vi "SEA_9811_Read.vi"(8 "error in (no error)":errorcluster, 11 "SEA9811_RT_data in":T2 {"Tx"."Tx Refs (Data,Trig)"."Data Reference" format="%.0x"}) -> (0 "error out":errorcluster, 1 "Receiver Status Register (RSR)":T1={"RSR0: FIFO channel 0 empty"=TRUE, "RSR1: FIFO channel 1 empty"=TRUE, "RSR2: FIFO channel 2 empty"=TRUE, "RSR3: FIFO channel 3 empty"=TRUE, "RSR4: FIFO channel 4 empty"=TRUE, "RSR5: FIFO channel 5 empty"=TRUE, "RSR6: FIFO channel 6 empty"=TRUE, "RSR7: FIFO channel 7 empty"=TRUE, "RSR8: FIFO channel 0 full"=FALSE, "RSR9: FIFO channel 1 full"=FALSE, "RSR10: FIFO channel 2 full"=FALSE, "RSR11: FIFO channel 3 full"=FALSE, "RSR12: FIFO channel 4 full"=FALSE, "RSR13: FIFO channel 5 full"=FALSE, "RSR14: FIFO channel 6 full"=FALSE, "RSR15: FIFO channel 7 full"=FALSE}, 3 "SEA9811_RT_data out":T2 {"Tx"."Tx Refs (Data,Trig)"."Data Reference" format="%.0x"}, 5 "DMA Overflow":bool)   [LabVIEW 2012]
doc: "Read words from FPGA, process and sync clock"
uses:
  Typdefs/SEA9811_RT_data_cluster.ctl
  <userlib>/_FPGA Interface Advanced Tools/FPGA Interface Base/FPGA Interface Base.lvclass
  Typdefs/FPGA ref.ctl
  Typdefs/channel.ctl
  Typdefs/received word.ctl
  Typdefs/SEA9811_FPGA_FP_Addresses.ctl
  <vilib>/NI Veristand/Custom Device API/Block Data Reference.ctl
  <vilib>/NI Veristand/Custom Device API/Data Reference.ctl
  FPGA/SEA-9811_ReceiverAndTransmitter/SubVIs/SEA-9811_ReceiverAndTransmitter_RSR.ctl
  <userlib>/_FPGA Interface Advanced Tools/FPGA Interface Wrapper/NiFPGA Read - U32.vi
  <userlib>/_FPGA Interface Advanced Tools/FPGA Interface Wrapper/NiFPGA Read - Boolean.vi
  <userlib>/_FPGA Interface Advanced Tools/FPGA Interface Wrapper/NiFPGA Read FIFO - U64.vi
  <userlib>/_FPGA Interface Advanced Tools/FPGA Interface Wrapper/NiFPGA Read - U16.vi
  <userlib>/_FPGA Interface Advanced Tools/FPGA Interface Wrapper/FPGA Interface Wrapper.lvlib
  <vilib>/NI Veristand/Custom Device API/Custom Device API.lvlib
panel:
  out "Elements Remaining":u32
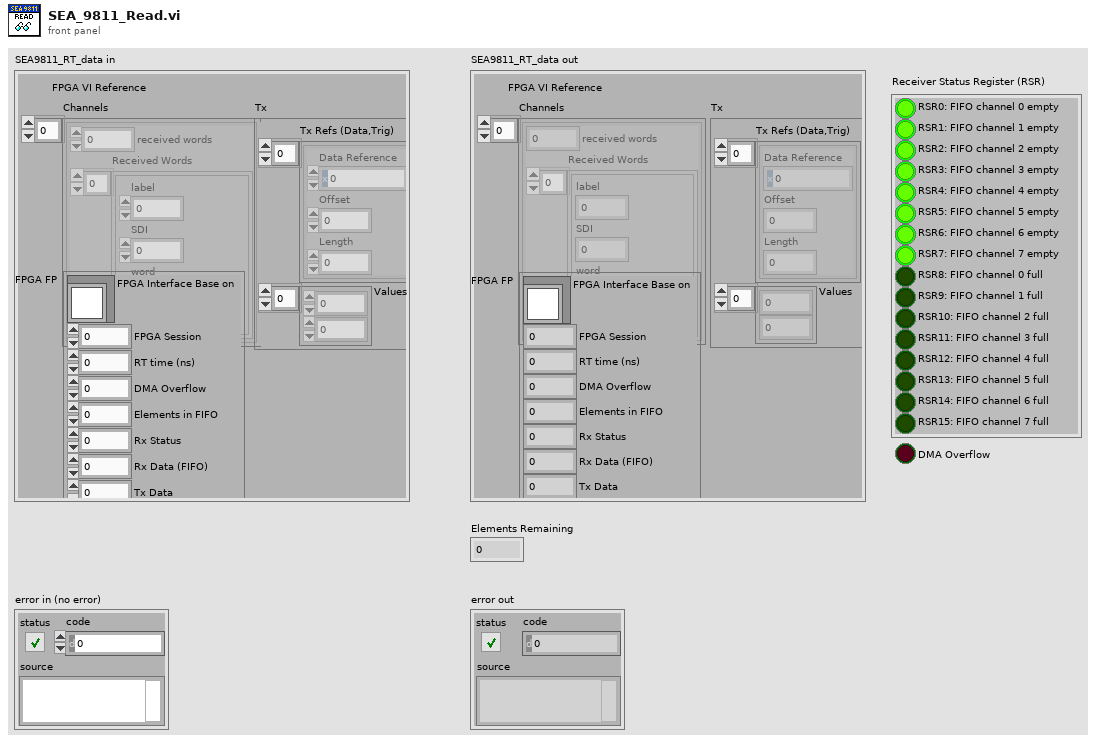
[diagram p1: front panel]
types:
  T1 = typedef "SEA-9811_ReceiverAndTransmitter_RSR.ctl" = cluster{"RSR0: FIFO channel 0 empty":bool, "RSR1: FIFO channel 1 empty":bool, "RSR2: FIFO channel 2 empty":bool, "RSR3: FIFO channel 3 empty":bool, "RSR4: FIFO channel 4 empty":bool, "RSR5: FIFO channel 5 empty":bool, "RSR6: FIFO channel 6 empty":bool, "RSR7: FIFO channel 7 empty":bool, "RSR8: FIFO channel 0 full":bool, "RSR9: FIFO channel 1 full":bool, "RSR10: FIFO channel 2 full":bool, "RSR11: FIFO channel 3 full":bool, "RSR12: FIFO channel 4 full":bool, "RSR13: FIFO channel 5 full":bool, "RSR14: FIFO channel 6 full":bool, "RSR15: FIFO channel 7 full":bool}
  T2 = typedef "SEA9811_RT_data_cluster.ctl" = cluster{"FPGA VI Reference":T3, "Channels":T4[], "FPGA FP":T6, "Tx":cluster{"Tx Refs (Data,Trig)":T7[], "Values":dbl[]}}
  T3 = typedef "FPGA ref.ctl" = refnum<k20>
  T4 = typedef "channel.ctl" = cluster{"received words":u32, "Received Words":T5[]}
  T5 = typedef "received word.ctl" = cluster{"label":u8, "SDI":u8, "word":u32, "timestamp":dbl}
  T6 = typedef "SEA9811_FPGA_FP_Addresses.ctl" = cluster{"FPGA Interface Base on":refnum<class "FPGA Interface Base.lvclass">, "FPGA Session":u32, "RT time (ns)":u32, "DMA Overflow":u32, "Elements in FIFO":u32, "Rx Status":u32, "Rx Data (FIFO)":u32, "Tx Data":u32, "Transmit Data":u32}
  T7 = typedef "Custom Device API.lvlib/Block Data Reference.ctl" = cluster{"Data Reference":T8, "Offset":i32, "Length":i32}
  T8 = typedef "Custom Device API.lvlib/Data Reference.ctl" = i32
  T9 = cluster{"Boolean array[0]":bool, "Boolean array[1]":bool, "Boolean array[2]":bool, "Boolean array[3]":bool, "Boolean array[4]":bool, "Boolean array[5]":bool, "Boolean array[6]":bool, "Boolean array[7]":bool, "Boolean array[8]":bool, "Boolean array[9]":bool, "Boolean array[10]":bool, "Boolean array[11]":bool, "Boolean array[12]":bool, "Boolean array[13]":bool, "Boolean array[14]":bool, "Boolean array[15]":bool}
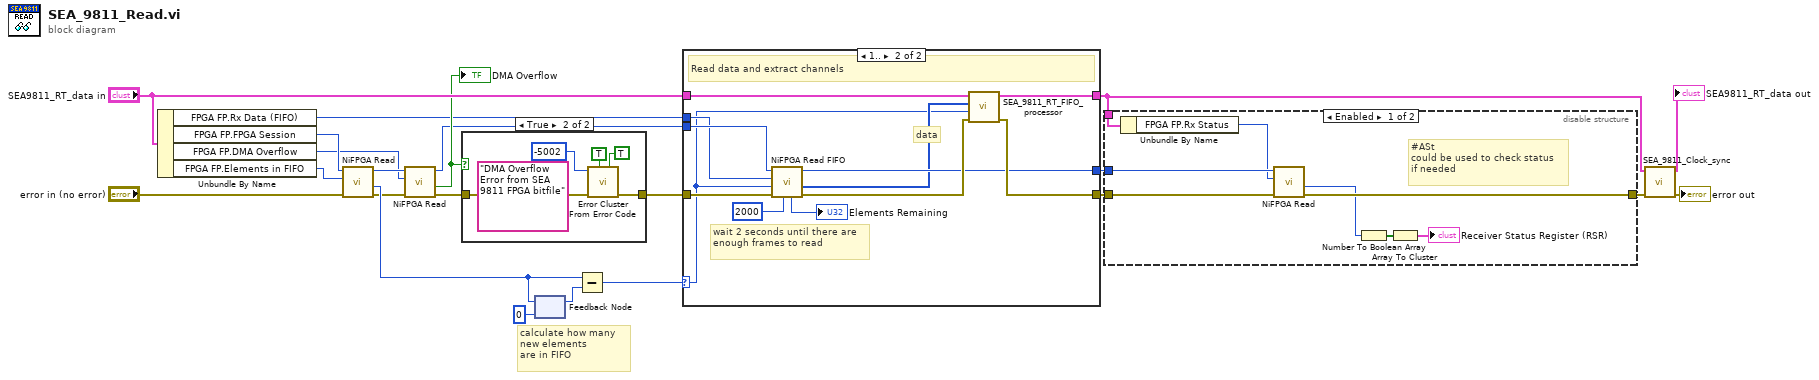
[diagram p0: block diagram]
diagram:
  # "calculate how many \nnew elements \nare in FIFO"
  n1 = Unbundle By Name("SEA9811_RT_data in") -> ("FPGA FP.Rx Data (FIFO)"=w6:u32, "FPGA FP.FPGA Session"=w17:u32, "FPGA FP.DMA Overflow"=w11:u32, "FPGA FP.Elements in FIFO"=w16:u32)
  n2 = call-poly <userlib>:"NiFPGA Read.vi"("error in (no error)"="error in (no error)", "Indicator"=w16, "Session"=w17) -> ("error out"=w12:errorcluster, "Value"=w14:u32, "Session Out"=w13:u32)  [unwired: 6 in]
  n3 = call-poly <userlib>:"NiFPGA Read.vi"("error in (no error)"=w12, "Indicator"=w11, "Session"=w13) -> ("error out"=w10:errorcluster, "Boolean"=w8:bool, "Session Out"=w7:u32)  [unwired: 6 in]
  "DMA Overflow" <- w8
  n4 = case shown="True" w8 {
    tunnel: w10 -> [w23 w29]
    tunnel: [w23 w28] -> w9
    frame False {
    }
    frame True {
      n5 = call <vilib>:"Error Cluster From Error Code.vi"("is warning? (False)"=TRUE, "show call chain? (False)"=TRUE, "error in (no error)"=w29, "error message (\"\")"="DMA Overflow Error from SEA 9811 FPGA bitfile" ("error message (\"\")"), "error code (0)"=-5002) -> ("error out"=w28:errorcluster)  [unwired: 4 in]
    }
  }
  n6 = feedback-in #1(w14) -> ()
  n7 = feedback #1(u32 0 ("Elements in FIFO")) -> (w22:u32)
  n8 = Subtract(x=w14, y=w22) -> (x-y=w1:u32)
  n9 = case shown="1.." w1 {
    selector: w1 -> [_ w33]
    tunnel: [w31 w42] -> w4
    tunnel: "SEA9811_RT_data in" -> [w32 w44]
    tunnel: [w32 w43] -> w5
    tunnel: w9 -> [w31 w40]
    tunnel: w7 -> [w30 w41]
    tunnel: w6 -> [_ w38]
    tunnel: [w30 w37] -> w2
    frame Default {
      # "not enough data to read"
    }
    frame 1.. {
      # "wait 2 seconds until there are enough frames to read"
      # "data"
      # "Read data and extract channels"
      n10 = call-poly <userlib>:"NiFPGA Read FIFO.vi"("Timeout"=u32 2000, "error in (no error)"=w40, "Number of Elements"=w33, "FIFO"=w38, "Session"=w41) -> ("error out"=w39:errorcluster, "Data"=w34:u64[], "Session Out"=w37:u32, "Elements Remaining"=→"Elements Remaining":u32)  [unwired: 3 in]
      n11 = call "SEA_9811_RT_FIFO_processor.vi"("error in (no error)"=w39, "Number of Elements"=w33, "9811 Data in"=w34, "SEA9811_RT_data in"=w44) -> ("error out"=w42:errorcluster, "SEA9811_RT_data out"=w43:T2)  [unwired: 6 in]
    }
  }
  n12 = disable-structure shown="Enabled" {
    disable-tunnel: w5 -> [w50 _]
    disable-tunnel: w4 -> [w49 w53]
    disable-tunnel: [w48 w53] -> w3
    disable-tunnel: w2 -> [w47 _]
    frame Enabled {
      # "#ASt\ncould be used to check status\nif needed"
      n13 = Unbundle By Name(w50) -> ("FPGA FP.Rx Status"=w46:u32)
      n14 = call-poly <userlib>:"NiFPGA Read.vi"("error in (no error)"=w49, "Indicator"=w46, "Session"=w47) -> ("error out"=w48:errorcluster, "Value"=w45:u16)  [unwired: 6 in, 1 out]
      n15 = Number To Boolean Array(number=w45) -> (Boolean array=w52:bool[])
      n16 = Array To Cluster(array=w52) -> (cluster=→"Receiver Status Register (RSR)":T9)
    }
    frame Disabled {
    }
  }
  n17 = call "SEA_9811_Clock_sync.vi"("error in (no error)"=w3, "SEA9811_RT_data in"=w5) -> ("error out"=→"error out":errorcluster, "SEA9811_RT_data out"=→"SEA9811_RT_data out":T2)  [unwired: 8 in]
